vi "SaveGestureState.vi"(11 "State":i32(ring)=-1 items=["STATESTART"=1, "STATEUPDATE"=2, "STATESTOP"=3, "STATEINVALID"=-1]) -> (3 "gesture state":T1)   [LabVIEW 2011, in "LMH-Leap.lvlib"]
uses:
  LMH-Leap.lvlib
  Type Defs/Gesture State.ctl
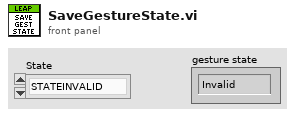
[diagram p1: front panel]
types:
  T1 = typedef "LMH-Leap.lvlib/Gesture State.ctl" = enum16{"Invalid", "Start", "Update", "Stop"}
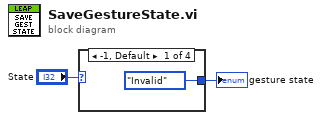
[diagram p0: block diagram]
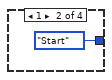
[diagram p2: hidden frame]
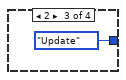
[diagram p3: hidden frame]
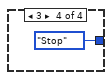
[diagram p4: hidden frame]
diagram:
  n1 = case shown="-1, Default" "State" {
    tunnel: [Gesture_State."Invalid" ("gesture state") Gesture_State."Start" ("gesture state") Gesture_State."Update" ("gesture state") Gesture_State."Stop" ("gesture state")] -> w2
    frame -1, Default {
    }
    frame 1 {
    }
    frame 2 {
    }
    frame 3 {
    }
  }
  "gesture state" <- w2
